vi "AlliGator Save-Load IRFs & Fit Data (Map).vi"(8 "error in (no error)":errorcluster, 9 "Write(T)/Load (F)":bool, 10 "File Path":path, 11 "Data Value Reference in":refnum<data-value>) -> (0 "error out":errorcluster, 3 "Data Value Reference out":refnum<data-value>, 4 "Message":string)   [LabVIEW 2021, in "AlliGator Decay Fit Parameter Map.lvlib"]
doc: "Load/Save Decay Fit Parameter Map & Metadata from/to HDF5 file."
uses:
  AlliGator Decay Fit Parameter Map.lvlib
  Internal Variables/AlliGator Internal Variables v2.ctl
  <vilib>/vision/Image Controls.llb/IMAQ Image.ctl
  Internal Variables/AlliGator Gate Image Set.ctl
  Files/AlliGator FLI Dataset Type.ctl
  Files/AlliGator Data Series Type.ctl
  Dual-Channel Datasets/AlliGator Dataset Channel.ctl
  Settings/AlliGator Gate Arithmetic.ctl
  Source Image/AlliGator Displayed Image.ctl
  Image/Named ROI Description.ctl
  Phasor Graph/AlliGator Decay Metadata v3.ctl
  Decay Analysis/Decay Preprocessing/AlliGator Decay Background Subtraction Info.ctl
  Decay Analysis/Decay Preprocessing/AlliGator Baseline Subtraction Method.ctl
  Graphs/XY Graph/XY Graph Plot Shift Parameters.ctl
  Graphs/XY Graph/XY Graph Plot Shift Method.ctl
  Decay Analysis/Decay Preprocessing/AlliGator Decay Extrapolation Parameters.ctl
  Phasor/Calibration Phasor (m, phi).ctl
  Phasor/Phasor Reference Series.ctl
  Phasor/Phasor Calibration Map v2.ctl
  Phasor/Phasor (g, s).ctl
  Phasor Graph/AlliGator Raw Phasor Plot Data v5.ctl
  Phasor/Phasor Standard Deviation Options.ctl
  Phasor Plot/AlliGator Phasor Multi-Harmonic Data.ctl
  Phasor/Phasor Harmonic Data.ctl
  AlliGator Decay Fit Options & Parameters v4.ctl
  Fits/IRF(X)PSED/Decay Fit Options v4.ctl
  Fits/Decay Convolution/Decay Model.ctl
  Fits/Residual Type.ctl
  Fits/IRF(X)PSED/Fit Weights Type v2.ctl
  Fits/Non-linear Fitting Method v2.ctl
  Fits/Fit Calculation Method.ctl
  Fits/Non-linear Fitting Algorithm.ctl
  Decay Analysis/Decay Fit/AlliGator Decay Fit Parameter Constraints 2.ctl
  Fits/IRF(X)PSED/Decay Fit Parameters In List.ctl
  Fits/IRF(X)PSED/MLE Baseline Offset Type.ctl
  Decay Analysis/Decay Preprocessing/AlliGator Decay Preprocessing Parameters.ctl
  Fits/IRF(X)PSED/Decay Fit Parameters & Derived Quantities List v2.ctl
  Fits/IRF(X)PSED/Decay Fit Result Constraint.ctl
  AlliGator Parameter Maps Data.ctl
  AlliGator IRFs & Fit Data v3.ctl
  Globals, Variables, Constants/AlliGator Globals.vi
  Files/AlliGator Files.lvlib
  Fits/Fits.lvlib
  Globals, Variables, Constants/AlliGator Globals, Variables & Constants.lvlib
  Graphs/XY Graph/XY Graph Add-Ons.lvlib
  Decay Analysis/Decay Preprocessing/AlliGator Decay Preprocessing.lvlib
  Phasor/Phasor.lvlib
  Image/Image.lvlib
  Phasor Graph/AlliGator Phasor Graph.lvlib
  Phasor Plot/AlliGator Phasor Plot.lvlib
  Source Image/AlliGator Source Image.lvlib
  Internal Variables/AlliGator Internal Variables.lvlib
  Decay Analysis/Decay Fit/AlliGator Decay Fit.lvlib
  Settings/AlliGator Settings.lvlib
  Dual-Channel Datasets/AlliGator Dual-Channel Datasets.lvlib
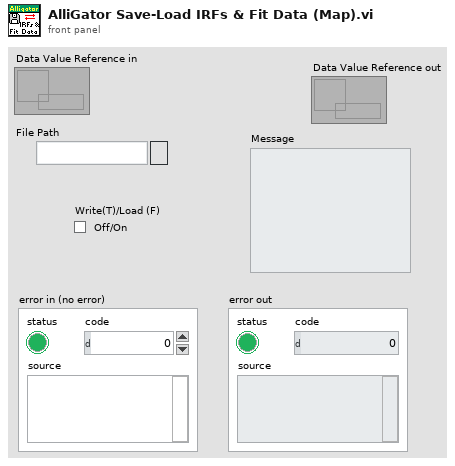
[diagram p1: front panel]
types:
  T1 = typedef "Fits.lvlib/Decay Model.ctl" = enum16{"1-Exponential", "2-Exponentials"}
  T2 = typedef "AlliGator Decay Fit Parameter Map.lvlib/AlliGator IRFs & Fit Data v3.ctl" = cluster{"IRF Array Time Axis":dbl[], "[IRFs]":dbl[][], "[Decay Fit Parameter Names]":T3[], "[Multiple Decays Fit Parameters]":dbl[][], "Fit Options: Decay Preprocessing Parameters":T4, "Fit Options: Reference Decay":cluster{"t Array":dbl[], "I Array":dbl[]}, "[Decay Sum]":dbl[]}
  T3 = typedef "Fits.lvlib/Decay Fit Parameters & Derived Quantities List v2.ctl" = enum16{"Offset", "Baseline", "A_1", "tau_1", "A_2", "tau_2", "<tau>_a", "f1_a", "f2_a", "<tau>_i", "f1_i", "f2_i", "-", "R^2", "Chi^2"}
  T4 = typedef "AlliGator Decay Preprocessing.lvlib/AlliGator Decay Preprocessing Parameters.ctl" = cluster{"Background Subtraction":bool, "Straighten Decay":bool, "Reverse Gates":bool, "1-Normalized Decay":bool, "Smoothen Decay":bool, "Smoothing Parameter":dbl, "Shift Decay":bool, "Decay Shift Parameters":T5, "Extrapolate Decay":bool, "Additional Points":u32, "Head Fraction":dbl, "Pixel-Normalize Decay":bool, "Use Periodicity":bool, "Use Cursors":bool, "Tail Fraction":dbl, "Use Decay Pre-Processing":bool, "Fold Decay":bool, "# Folds":u32, "[0-1]-Normalized Decay":bool}
  T5 = typedef "XY Graph Add-Ons.lvlib/XY Graph Plot Shift Parameters.ctl" = cluster{"Type":T6, "Shift":dbl[unit], "Threshold":dbl, "Rotate":bool}
  T6 = typedef "XY Graph Add-Ons.lvlib/XY Graph Plot Shift Method.ctl" = enum16{"Default", "CFD", "Threshold", "Cross-Correlation"}
  T7 = typedef "AlliGator Internal Variables.lvlib/AlliGator Internal Variables v2.ctl" = cluster{"----------------------------- Images -----------------------------":u8, "Displayed Image":T8, "White Light Image":T8, "Mask Image":T8, "ROI Mask Image":T8, "Current Dataset Images 1":T9, "Background Dataset Images 1":T9, "Current Dataset Images 2":T9, "Background Dataset Images 2":T9, "Current Dataset Arithmetic Images":T9, "Accumulated Dataset Images 1":T9, "Accumulated Dataset Images 2":T9, "Accumulated Dataset Arithmetic Images":T9, "----------------------------- File Paths -----------------------------":u8, "Phasor Plot Image":T8, "Decay Fit Parameter Map Image":T8, "Parameter Map Image":T8, "Single Data Point Path":path, "White Light Image Path":path, "Mask Image Path":path, "Time-Series Folder":path, "[Time-Series Paths]":path[], "----------------------------- FLI Dataset -----------------------------":u8, "Current Dataset":i32, "Single Dataset Type":T10, "Current Folder":string, "AlliGator Data Series Type":T11, "# Datasets":i32, "Dual-Channel Dataset":bool, "Selected Channel Name":string, "Dataset Channel":T12, "Channel Arithmetic":T13, "Dual-Channel Background Dataset":bool, "Background Channel":T12, "Dual-Channel Accumulated Dataset":bool, "Start Time":dbl, "[Time-Series Timestamps]":dbl[], "[Intensity Corrections]":dbl[], "Time Series Script":bool, "Type of Displayed Image":T14, "Gate Image Slide":u16, "# Gates":i32, "ROIs":T15[], "----------------------------- Decays -----------------------------":u8, "ROI Decay":cluster{"t Array":dbl[], "I Array":dbl[]}, "Valid Decay":bool, "Decay  Metadata":T17, "Reference Decay Plot Name":string, "Reference Decay":cluster{"t Array":dbl[], "I Array":dbl[]}, "Decay Shift Plot":cluster{"Time Stamps":dbl[], "Decay Shifts":dbl[]}, "[Decays Max Values]":sgl[], "[Decays Min Values]":sgl[], "----------------------------- Calibration -----------------------------":u8, "Calibration Phasor":T21, "Calibration Phasor Series":T22, "Phasor Calibration Map":T23, "Calibration Map MD5 Digest":string, "----------------------------- Phasor Graph -----------------------------":u8, "Last Raw Phasor":T24, "Last Calibrated Phasor":T24, "Last Calibrated Phasor SDV":T24, "Phasor Graph:Phasor Plot":cluster{"g Array":dbl[], "s Array":dbl[]}, "Phasor Graph:Phasor SDV Plot":cluster{"g Array":dbl[], "s Array":dbl[]}, "[Phasor Graph:Raw Phasor Plots]":T25[], "Phasor Plot locked to Ref 1":i32, "[Phasor Plot(s) locked to Ref 1]":i32[], "[Phasor Plot(s) locked to Ref 2]":i32[], "[Pixel Phasors]":T24[], "----------------------------- Phasor Plot -----------------------------":u8, "[[Sum Image]]":dbl[][], "[[CSG Phasors]]":csg[][], "[[Valid Pixel?]]":bool[][], "[[Phasor Ratios]]":dbl[][], "[[Average Lifetimes]]":dbl[][], "Amplitude Weighted Average Lifetime":bool, "I/m/phi Dataset":cluster{"I/m/phi Dataset?":bool, "Base Frequency":dbl[unit], "Harmonic Orders":u8[]}, "Multi Phasor Plot Data":T27, "----------------------------- Decay Fit Parameter Map -----------------------------":u8, "Decay Fit Options & Parameters":T29, "Fit Options: Decay Preprocessing Parameters":T4, "Fit Options: Reference Decay":cluster{"t Array":dbl[], "I Array":dbl[]}, "Is Full Image Parameters Map":bool, "Is Single-Pixels Parameters Map":bool, "NLSF Parameters Map X Resolution":i32, "NLSF Parameters Map Y Resolution":i32, "[Single Decay Fit Parameters]":dbl[], "Fit Model":T1, "[[Multiple Decays Fit Parameters]]":dbl[][], "[[Multiple Decays Fit Parameter SDVs]]":dbl[][], "[[IRFs]]":dbl[][], "[ROI Descriptors]":T16[], "IRF Array Time Axis":dbl[], "Decay Array Time Axis":dbl[], "[Decay Fit Parameter Names]":T3[], "[Decay Sum]":dbl[], "Array of Decay Fit Result Constraints":T39[], "Selected ROIs Array":bool[], "----------------------------- Parameter Maps -----------------------------":u8, "[Map Set Names]":string[], "[Parameter Maps]":T40[], "[[User-defined Quantities]]":dbl[][], "User-defined Quantity":string}
  T8 = typedef "IMAQ Image.ctl" = refnum<image>
  T9 = typedef "AlliGator Internal Variables.lvlib/AlliGator Gate Image Set.ctl" = cluster{"SGL Image Max":T8, "SGL Image Sum":T8, "SGL Gate Images":T8[], "SGL Image Min":T8}
  T10 = typedef "AlliGator Files.lvlib/AlliGator FLI Dataset Type.ctl" = enum16{"HDF5 FLI Dataset", "Gate Image Folder", ".sdt FLI Dataset (Becker & Hickl)", ".ptu FLI Dataset (PicoQuant)", "SS1 FLI Dataset", "SS2 FLI Dataset", "I/m/phi Dataset", ".bin FLI Dataset (PicoQuant Binned)", ".bin FLI Dataset (Piccolo Binned)", ".mat FLI Dataset"}
  T11 = typedef "AlliGator Files.lvlib/AlliGator Data Series Type.ctl" = enum16{"Not a Supported Series", "Gate Images Folder Series", "SwissSPAD 2 Dataset Series", "B&H FLI Dataset Series", "PicoQuant PTU FLI Dataset Series", "PicoQuant BIN FLI Dataset Series", "Piccolo hist BIN FLI Dataset Series", "HDF5 FLI Dataset Series"}
  T12 = typedef "AlliGator Dual-Channel Datasets.lvlib/AlliGator Dataset Channel.ctl" = enum16{"G2", "INT"}
  T13 = typedef "AlliGator Settings.lvlib/AlliGator Gate Arithmetic.ctl" = enum16{"None", "INT-G2", "G2/INT*<INT>", "(1 - G2/INT)*<INT>"}
  T14 = typedef "AlliGator Source Image.lvlib/AlliGator Displayed Image.ctl" = enum16{"Single Gate", "Sum of All Gates", "Max of All Gates", "Min of All Gates", "-", "White Ligth Image", "Mask Image"}
  T15 = typedef "Image.lvlib/Named ROI Description.ctl" = cluster{"ROI Descriptor":T16, "ROI Name":string, "Overlay Color":u32}
  T16 = typedef "ROI Descriptor" = cluster{"Global Rectangle":i32[], "Contours":cluster{"ID":enum32{"External", "Internal"}, "Type":u32, "Coordinates":i32[]}[]}
  T17 = typedef "AlliGator Phasor Graph.lvlib/AlliGator Decay Metadata v3.ctl" = cluster{"ROI Descriptor":T16, "ROI Center":cluster{"X":i32, "Y":i32}, "Decay Background Subtraction Info":T18, "Decay Reverted":bool, "Decay Smoothened":bool, "Decay Straightened":bool, "Fitted Tau (Decay Straightening)":dbl, "Decay Shift Parameters":T5, "Decay Shifted":bool, "Decay Extrapolated":bool, "Decay Extrapolation Parameters":T20, "Decay Normalized":bool, "Fold Decay":bool, "# Folds":u32}
  T18 = typedef "AlliGator Decay Preprocessing.lvlib/AlliGator Decay Background Subtraction Info.ctl" = cluster{"Laser Period":dbl[unit], "Gate Duration":dbl[unit], "Baseline Subtraction Method":T19, "Background Definition Range":cluster{"Min Gate":dbl[unit], "Max Gate":dbl[unit]}, "Total Intensity w/o Bkgd Subtraction":dbl, "Bkgd-subtracted Intensity (exp)":dbl, "# Data Points":i32, "Background/Gate":dbl, "Fitted Lifetime":dbl[unit], "Bkgd-subtracted Intensity (theo)":dbl}
  T19 = typedef "AlliGator Decay Preprocessing.lvlib/AlliGator Baseline Subtraction Method.ctl" = enum16{"Mean", "Min", "Square Gated Single-Exponential", "File", "Constant"}
  T20 = typedef "AlliGator Decay Preprocessing.lvlib/AlliGator Decay Extrapolation Parameters.ctl" = cluster{"Additional Points":u32, "Head Fraction":dbl, "Fitted Tau":dbl, "Use Periodicity":bool, "Use Cursors":bool, "Tail Fraction":dbl}
  T21 = typedef "Phasor.lvlib/Calibration Phasor (m, phi).ctl" = cluster{"m":dbl, "phi":dbl, "Phasor Frequency":dbl[unit], "Reference Lifetime":dbl[unit]}
  T22 = typedef "Phasor.lvlib/Phasor Reference Series.ctl" = cluster{"m Array":dbl[], "phi Array":dbl[], "Phasor Frequency":dbl[unit], "Calibration Lifetime":dbl[unit]}
  T23 = typedef "Phasor.lvlib/Phasor Calibration Map v2.ctl" = cluster{"Phasor Frequency":dbl[unit], "Calibration Lifetime":dbl[unit], "ROI Centers":cluster{"X":i32, "Y":i32}[], "ROI Descriptors":T16[], "Map Resolution X":i32, "Map Resolution Y":i32, "z Array":cdb[]}
  T24 = typedef "Phasor.lvlib/Phasor (g, s).ctl" = cluster{"g":dbl, "s":dbl}
  T25 = typedef "AlliGator Phasor Graph.lvlib/AlliGator Raw Phasor Plot Data v5.ctl" = cluster{"Phasor Plot Name":string, "Raw Phasor Plot":T24[], "Phasor Frequency":dbl[unit], "[Decay Metadata]":T17[], "Raw Phasor Plot SDV":T24[], "Phasor SDV Options":T26, "[Calibration Phasor]":T21[], "Intensity Array":dbl[]}
  T26 = typedef "Phasor.lvlib/Phasor Standard Deviation Options.ctl" = cluster{"Compute Estimated SDV":bool, "# Replicas":u32, "Use Estimated Average Phasor":bool}
  T27 = typedef "AlliGator Phasor Plot.lvlib/AlliGator Phasor Multi-Harmonic Data.ctl" = cluster{"Base Frequency":dbl[unit], "# Harmonics":u8, "Harmonic Orders":u8[], "Phasor Plot Settings Checksum":u64, "Phasor Harmonic Data Array":T28[]}
  T28 = typedef "Phasor.lvlib/Phasor Harmonic Data.ctl" = cluster{"Phasor Harmonic Name":string, "Phasor Plot Settings Checksum":u64, "Phasor Frequency":dbl[unit], "Base Frequency":dbl[unit], "Harmonic Order":u8, "Phasor Plot Parameters":string, "Phasor Array [[CSG]]":csg[][], "Dataset File Path":path}
  T29 = typedef "AlliGator Decay Fit Parameter Map.lvlib/AlliGator Decay Fit Options & Parameters v4.ctl" = cluster{"SYNC Period":dbl[unit], "Fit Options":T30, "Fit Parameter Constraints":T36[], "MLE Baseline Offset":dbl, "MLE Baseline Offset Type":T38}
  T30 = typedef "Fits.lvlib/Decay Fit Options v4.ctl" = cluster{"Show Fit Residuals":bool, "Fit Model":T1, "Residual Type":T31, "Max Decay Percentile":dbl, "Min Decay Percentile":dbl, "Show Full Decay":bool, "Weights":T32, "Fitting Method":T33, "Compute Parameter Uncertainties":bool, "Periodic Boundaries":bool, "Model Calculation":T34, "Period":dbl[unit], "Termination Criteria":cluster{"Max Iterations":i32, "Max Function Calls":i32, "Max Time":dbl[unit], "Function Tolerance":dbl, "Parameter Tolerance":dbl, "Gradient Tolerance":dbl, "Min Lambda":dbl, "Max Lambda":dbl, "Initial Tick Count":u32}, "Offset Resolution":dbl[unit], "Use Local IRF":bool, "Fitting Algorithm":T35, "Show Confidence Interval ":bool, "Confidence Level":dbl}
  T31 = typedef "Fits.lvlib/Residual Type.ctl" = enum16{"Standard", "Normalized", "Reduced"}
  T32 = typedef "Fits.lvlib/Fit Weights Type v2.ctl" = enum16{"Unweighted", "1/Variance (Neyman)", "1/Variance (Pearson)", "Best of All"}
  T33 = typedef "Fits.lvlib/Non-linear Fitting Method v2.ctl" = enum16{"Least Square", "Least Absolute Residual", "Bisquare", "MLE", "-", "Best of All"}
  T34 = typedef "Fits.lvlib/Fit Calculation Method.ctl" = enum16{"Simulation", "Convolution", "Integration"}
  T35 = typedef "Fits.lvlib/Non-linear Fitting Algorithm.ctl" = enum16{"Levenberg-Marquardt", "Trust-Region Dogleg"}
  T36 = typedef "AlliGator Decay Fit.lvlib/AlliGator Decay Fit Parameter Constraints 2.ctl" = cluster{"Fit Parameter":T37, "Min Value":dbl, "Max Value":dbl, "Global":bool, "Used":bool}
  T37 = typedef "Fits.lvlib/Decay Fit Parameters In List.ctl" = enum16{"Offset", "Baseline", "A_1", "tau_1", "A_2", "tau_2"}
  T38 = typedef "Fits.lvlib/MLE Baseline Offset Type.ctl" = enum32{"Absolute", "Percentage"}
  T39 = typedef "Fits.lvlib/Decay Fit Result Constraint.ctl" = cluster{"Fit Parameter":enum16{"Offset", "Baseline", "A_1", "tau_1", "A_2", "tau_2", "<tau>_a", "f1_a", "f2_a", "<tau>_i", "f1_i", "f2_i", "-", "R^2", "Chi^2", "Max Relative Residual", "<Residual ACF>", "Residual ACF SDV", "tau_2/tau_1"}, "Min Value":dbl, "Max Value":dbl, "Use Constraint":bool}
  T40 = typedef "AlliGator Decay Fit Parameter Map.lvlib/AlliGator Parameter Maps Data.ctl" = cluster{"Map Set Name":string, "[Parameter Names]":string[], "[[Parameters]]":dbl[][], "[[Parameter SDVs]]":dbl[][], "Decay Array Time Axis":dbl[], "[[IRFs]]":dbl[][], "IRF Array Time Axis":dbl[], "X Resolution":i32, "Y Resolution":i32, "Intensity Array":dbl[]}
  T41 = typedef "AlliGator Decay Fit Parameter Map.lvlib/AlliGator IRFs & Fit Data v1.ctl" = cluster{"IRF Array Time Axis":dbl[], "[IRF]":dbl[][], "[Decay Fit Parameter Name]":T3[], "[Multiple Decays Fit Parameters]":dbl[][]}
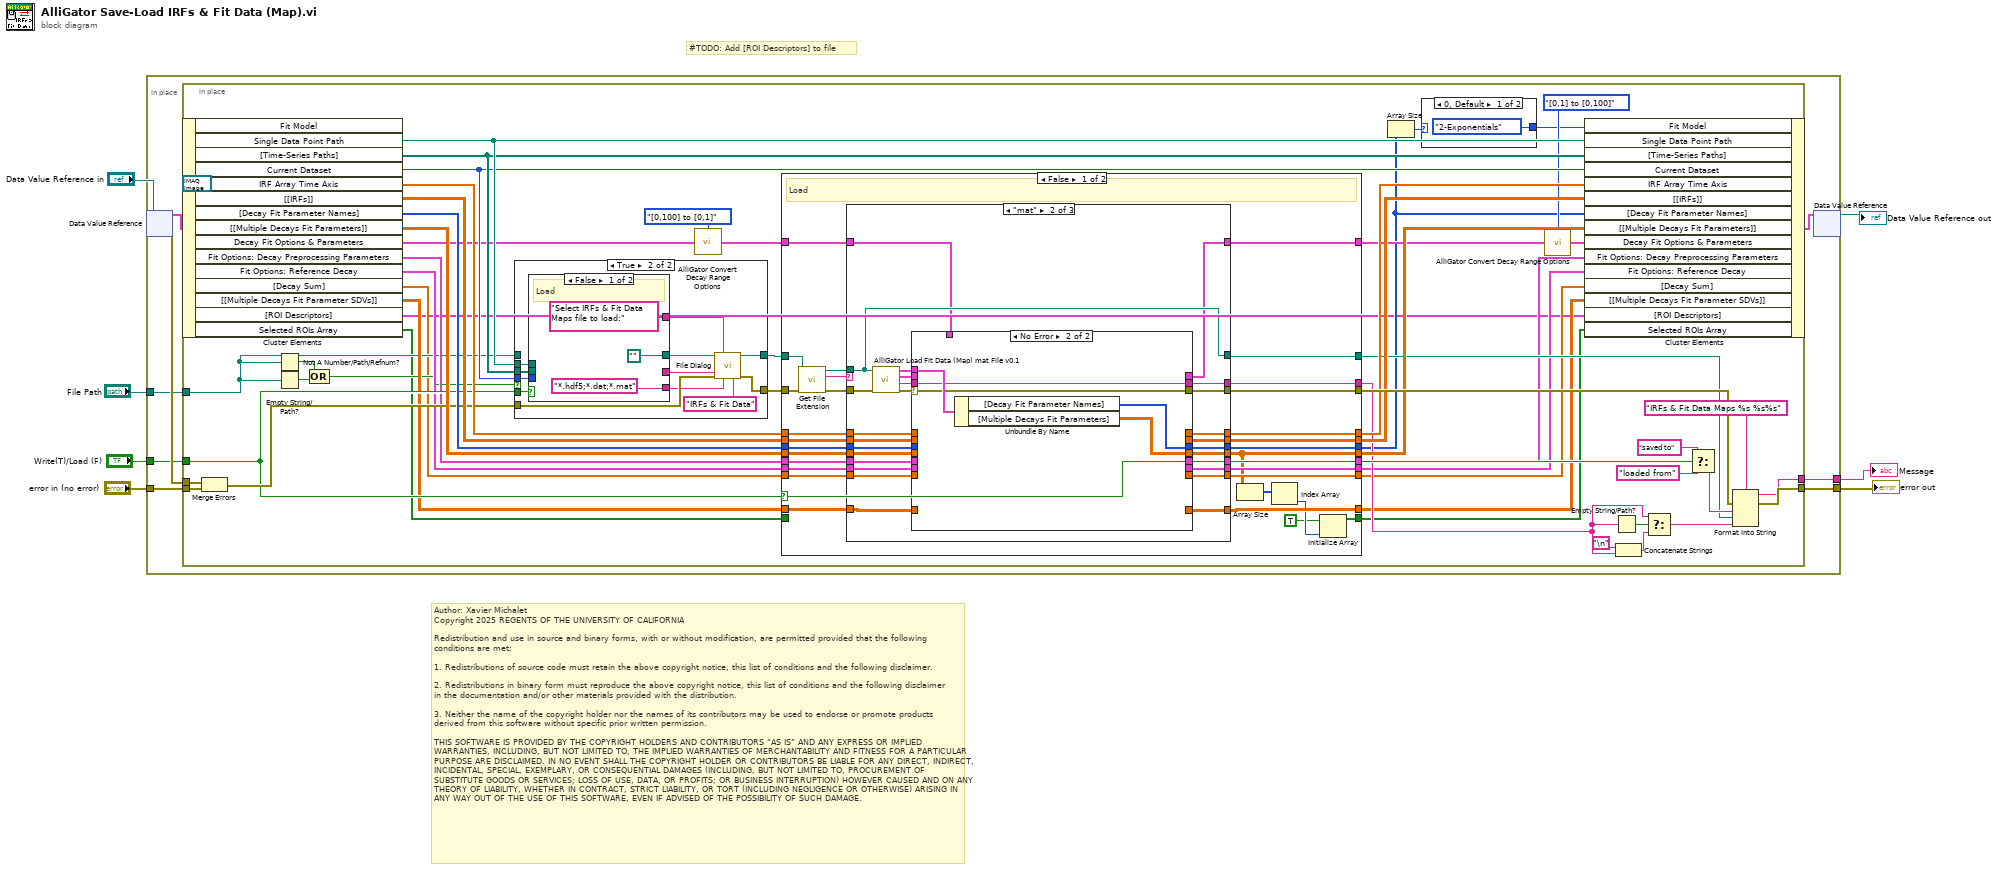
[diagram p0: block diagram]
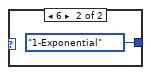
[diagram p2: hidden frame]
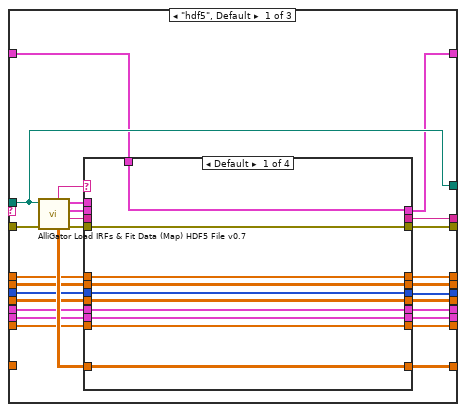
[diagram p3: hidden frame]
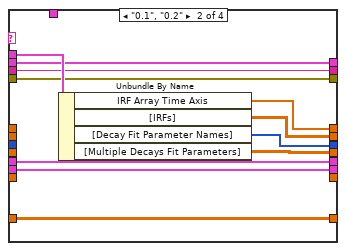
[diagram p4: hidden frame]
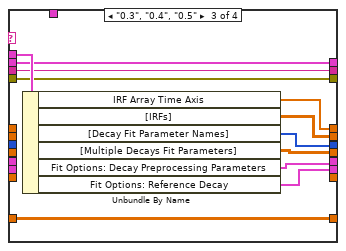
[diagram p5: hidden frame]
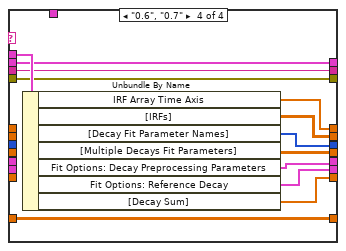
[diagram p6: hidden frame]
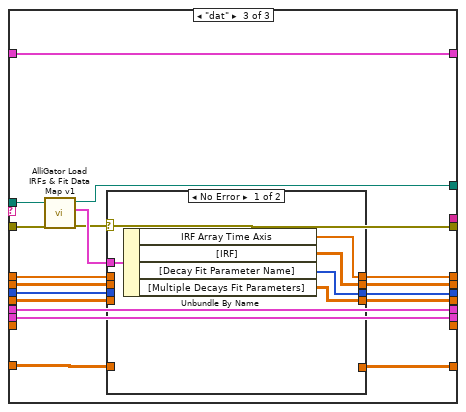
[diagram p8: hidden frame]
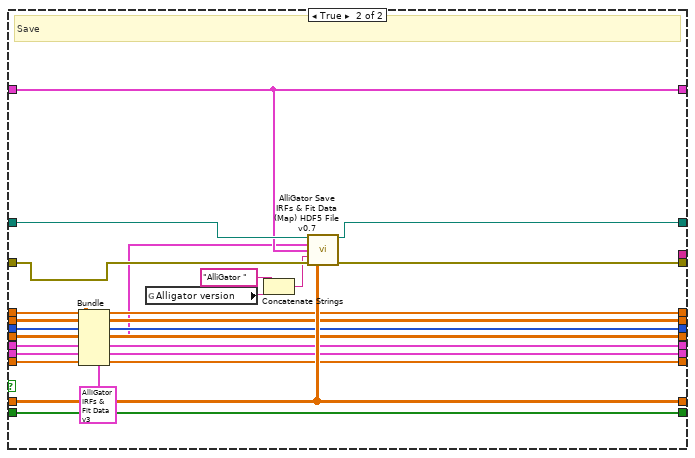
[diagram p10: hidden frame]
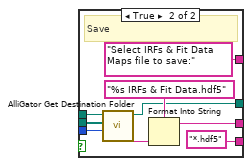
[diagram p12: hidden frame]
diagram:
  # "#TODO: Add [ROI Descriptors] to file"
  # "Author: Xavier Michalet\nCopyright 2025 REGENTS OF THE UNIVERSITY OF CALIFORNIA\n\nRedistribution and use in source and binary forms, with or without modification, are permitted provided that the following conditions are met:\n\n1. Redistributions of source code must retain the above copyright notice, this list of conditions and the following disclaimer.\n\n2. Redistributions in binary form must reproduce the above copyright notice, this list of conditions and the following disclaimer in the documentation and/or other materials provided with the distribution.\n\n3. Neither the name of the copyright holder nor the names of its contributors may be used to endorse or promote products derived from this software without specific prior written permission.\n\nTHIS SOFTWARE IS PROVIDED BY THE COPYRIGHT HOLDERS AND CONTRIBUTORS “AS IS” AND ANY EXPRESS OR IMPLIED WARRANTIES, INCLUDING, BUT NOT LIMITED TO, THE IMPLIED WARRANTIES OF MERCHANTABILITY AND FITNESS FOR A PARTICULAR PURPOSE ARE DISCLAIMED. IN NO EVENT SHALL THE COPYRIGHT HOLDER OR CONTRIBUTORS BE LIABLE FOR ANY DIRECT, INDIRECT, INCIDENTAL, SPECIAL, EXEMPLARY, OR CONSEQUENTIAL DAMAGES (INCLUDING, BUT NOT LIMITED TO, PROCUREMENT OF SUBSTITUTE GOODS OR SERVICES; LOSS OF USE, DATA, OR PROFITS; OR BUSINESS INTERRUPTION) HOWEVER CAUSED AND ON ANY THEORY OF LIABILITY, WHETHER IN CONTRACT, STRICT LIABILITY, OR TORT (INCLUDING NEGLIGENCE OR OTHERWISE) ARISING IN ANY WAY OUT OF THE USE OF THIS SOFTWARE, EVEN IF ADVISED OF THE POSSIBILITY OF SUCH DAMAGE."
  n1 = in-place {
    in-place-border: "error in (no error)" -> [w13]
    in-place-border: [w11] -> w1
    in-place-border: [w10] -> w2
    in-place-border: "Write(T)/Load (F)" -> [w9]
    in-place-border: "File Path" -> [w8]
    n2 = in-place-dvr #1("Data Value Reference in") -> (w15:T7, w12:errorcluster)
    n3 = in-place {
      in-place-border: w13 -> [w68]
      in-place-border: w12 -> [w64]
      in-place-border: [w62] -> w11
      in-place-border: [w61] -> w10
      in-place-border: w9 -> [w43]
      in-place-border: w8 -> [w23]
      (unwired) T8 refnum ("Current Dataset Images.Image Sum")
      n4 = in-place-cluster #2(w15) -> ("Single Data Point Path"=w67:path, "[Time-Series Paths]"=w66:path[], "Current Dataset"=w65:i32, "IRF Array Time Axis"=w56:dbl[], "[[IRFs]]"=w55:dbl[][], "[Decay Fit Parameter Names]"=w54:T3[], "[[Multiple Decays Fit Parameters]]"=w53:dbl[][], "Decay Fit Options & Parameters"=w44:T29, "Fit Options: Decay Preprocessing Parameters"=w35:T4, "Fit Options: Reference Decay"=w34:cluster{"t Array":dbl[], "I Array":dbl[]}, "[Decay Sum]"=w20:dbl[], "[[Multiple Decays Fit Parameter SDVs]]"=w37:dbl[][], "[ROI Descriptors]"=w18:T16[], "Selected ROIs Array"=w17:bool[])  [unwired: 1 out]
      n5 = Merge Errors(w64, w68) -> (w47:errorcluster)
      n6 = Not A Number/Path/Refnum?(number/path/refnum=w23) -> (NaN/Path/Refnum?=w21:bool)
      n7 = Empty String/Path?(string/path=w23) -> (empty?=w48:bool)
      n8 = Compound Arithmetic op=OR(w21, w48) -> (w22:bool)
      n9 = case shown="True" w22 {
        tunnel: w67 -> [_ w273]
        tunnel: w66 -> [_ w272]
        tunnel: w65 -> [_ w271]
        tunnel: w23 -> [w261 _]
        tunnel: w47 -> [w260 w268]
        tunnel: [w261 w267] -> w46
        tunnel: [w260 w266] -> w45
        tunnel: w43 -> [_ w264]
        frame False {
        }
        frame True {
          n10 = case shown="False" w264 {
            tunnel: w273 -> [_ w285]
            tunnel: w272 -> [_ w284]
            tunnel: w271 -> [_ w283]
            tunnel: [path "" w280] -> w270
            tunnel: [_ w279] -> w269
            tunnel: ["Select IRFs & Fit Data Maps file to load:" ("prompt") "Select IRFs & Fit Data Maps file to save:" ("prompt")] -> w263
            tunnel: ["*.hdf5;*.dat;*.mat" ("pattern (all files)") "*.hdf5" ("pattern (all files)")] -> w262
            frame False {
              # "Load"
            }
            frame True {
              # "Save"
              n11 = call "AlliGator Get Destination Folder.vi"("Current Data Set (-1: single)"=w283, "Time-Series Paths"=w284, "Single Data Point Path"=w285) -> ("Data Point Name"=w282:string, "Destination Folder path"=w280:path)  [unwired: 5 in, 2 out]
              n12 = Format Into String(format string="%s IRFs & Fit Data.hdf5", w282) -> (resulting string=w279:string)  [unwired: 2 in, 1 out]
            }
          }
          n13 = call "File Dialog"("start path"=w270, "prompt"=w263, "default name"=w269, "error in"=w268, "pattern (all files)"=w262, "pattern label"="IRFs & Fit Data") -> ("selected path"=w267:path, "error out"=w266:errorcluster)  [unwired: 6 in, 2 out]
        }
      }
      n14 = call "AlliGator Convert Decay Range Options.vi"("Decay Fit Options & Parameters in"=w44, "Percentile Conversion"=enum32{"[0,1] to [0,100]", "[0,100] to [0,1]"}."[0,100] to [0,1]") -> ("Decay Fit Options & Parameters out"=w31:T29)
      n15 = case shown="False" w43 {
        tunnel: [w93 w258] -> w63
        tunnel: [w92 w259] -> w49
        tunnel: w56 -> [w97 w253]
        tunnel: w55 -> [w96 w252]
        tunnel: w54 -> [w95 w251]
        tunnel: w53 -> [w94 w250]
        tunnel: [w100 w253] -> w52
        tunnel: [w99 w252] -> w51
        tunnel: [w98 w251] -> w26
        tunnel: [w75 w250] -> w50
        tunnel: w46 -> [w91 w257]
        tunnel: w45 -> [w89 w256]
        tunnel: w31 -> [w85 w255]
        tunnel: [w86 w255] -> w29
        tunnel: [w84 _] -> w40
        tunnel: w37 -> [w82 w254]
        tunnel: [w83 w254] -> w36
        tunnel: w35 -> [w81 w249]
        tunnel: w34 -> [w79 w248]
        tunnel: [w80 w249] -> w33
        tunnel: [w78 w248] -> w32
        tunnel: w20 -> [w76 w242]
        tunnel: [w77 w242] -> w19
        tunnel: w17 -> [_ w241]
        tunnel: [w71 w241] -> w16
        frame False {
          # "Load"
          n16 = call <vilib>:"Get File Extension.vi"("error in (no error)"=w89, "file"=w91) -> ("error out"=w90:errorcluster, "lowercase file extension"=w88:string, "dup file"=w87:path)  [unwired: 5 in, 2 out]
          n17 = case shown="\"mat\"" w88 {
            tunnel: [w125 w195 w229] -> w100
            tunnel: [w124 w194 w228] -> w99
            tunnel: [w123 w193 w227] -> w98
            tunnel: [w122 w192 w226] -> w75
            tunnel: w97 -> [w107 w179 w225]
            tunnel: w96 -> [w106 w178 w224]
            tunnel: w95 -> [w105 w177 w223]
            tunnel: w94 -> [w104 w176 w222]
            tunnel: [w120 w190 w221] -> w93
            tunnel: [w119 w189 w220] -> w92
            tunnel: w90 -> [w127 w197 w219]
            tunnel: w87 -> [w119 w189 w218]
            tunnel: [w114 w185 w217] -> w86
            tunnel: w85 -> [w103 w175 w217]
            tunnel: [w113 w184 _] -> w84
            tunnel: [w115 w186 w215] -> w83
            tunnel: w82 -> [_ w172 w216]
            tunnel: w81 -> [w111 w183 w214]
            tunnel: [w110 w182 w214] -> w80
            tunnel: w79 -> [w109 w181 w213]
            tunnel: [w108 w180 w213] -> w78
            tunnel: [w102 w174 _] -> w77
            tunnel: w76 -> [w101 w173 _]
            frame "hdf5", Default {
              n18 = call "AlliGator Load IRFs & Fit Data (Map) HDF5 File v0.7.vi"("Error In"=w127, "File Path"=w119) -> ("error out"=w121:errorcluster, "Data Description"=w117:string, "Decay Fit Options & Parameters"=w118:T29, "IRFs & Fit Data Map v3"=w126:T2, "[Multiple Decays Fit Parameters SDV]"=w116:dbl[][], "File Version"=w112:string)  [unwired: 3 in, 1 out]
              n19 = case shown="Default" w112 {
                tunnel: w126 -> [_ w148 w159 w171]
                tunnel: [w137 w147 w158 w170] -> w125
                tunnel: [w136 w146 w157 w169] -> w124
                tunnel: [w135 w145 w156 w168] -> w123
                tunnel: [w134 w144 w155 w167] -> w122
                tunnel: [w130 w143 w154 w166] -> w120
                tunnel: w118 -> [_ w141 w152 w165]
                tunnel: w117 -> [_ w140 w151 w164]
                tunnel: w116 -> [w131 w142 w153 w161]
                tunnel: [w131 w142 w153 w161] -> w115
                tunnel: [w129 w141 w152 w165] -> w114
                tunnel: [_ w140 w151 w164] -> w113
                tunnel: w121 -> [w130 w143 w154 w166]
                tunnel: [w133 w139 w150 w163] -> w110
                tunnel: w111 -> [w133 w139 _ _]
                tunnel: w109 -> [w132 w138 _ _]
                tunnel: [w132 w138 w149 w162] -> w108
                tunnel: w107 -> [w137 _ _ _]
                tunnel: w106 -> [w136 _ _ _]
                tunnel: w105 -> [w135 _ _ _]
                tunnel: w104 -> [w134 _ _ _]
                tunnel: w103 -> [w129 _ _ _]
                tunnel: [w128 _ _ w160] -> w102
                tunnel: w101 -> [w128 _ _ _]
                frame Default {
                }
                frame "0.1", "0.2" {
                  n20 = Unbundle By Name(w148) -> ("IRF Array Time Axis"=w147:dbl[], "[IRFs]"=w146:dbl[][], "[Decay Fit Parameter Names]"=w145:T3[], "[Multiple Decays Fit Parameters]"=w144:dbl[][])
                }
                frame "0.3", "0.4", "0.5" {
                  n21 = Unbundle By Name(w159) -> ("IRF Array Time Axis"=w158:dbl[], "[IRFs]"=w157:dbl[][], "[Decay Fit Parameter Names]"=w156:T3[], "[Multiple Decays Fit Parameters]"=w155:dbl[][], "Fit Options: Decay Preprocessing Parameters"=w150:T4, "Fit Options: Reference Decay"=w149:cluster{"t Array":dbl[], "I Array":dbl[]})
                }
                frame "0.6", "0.7" {
                  n22 = Unbundle By Name(w171) -> ("IRF Array Time Axis"=w170:dbl[], "[IRFs]"=w169:dbl[][], "[Decay Fit Parameter Names]"=w168:T3[], "[Multiple Decays Fit Parameters]"=w167:dbl[][], "Fit Options: Decay Preprocessing Parameters"=w163:T4, "Fit Options: Reference Decay"=w162:cluster{"t Array":dbl[], "I Array":dbl[]}, "[Decay Sum]"=w160:dbl[])
                }
              }
            }
            frame "mat" {
              n23 = call "AlliGator Load Fit Data (Map) mat File v0.1.vi"("Error In"=w197, "File Path"=w189) -> ("error out"=w191:errorcluster, "Data Description"=w187:string, "Decay Fit Options & Parameters"=w188:T29, "IRFs & Fit Data Map v3"=w196:T2)  [unwired: 3 in, 3 out]
              n24 = case shown="No Error" w191 {
                selector: w191 -> [w200 w209]
                tunnel: w196 -> [_ w212]
                tunnel: [w207 _] -> w195
                tunnel: [w206 _] -> w194
                tunnel: [w205 w211] -> w193
                tunnel: [w204 w210] -> w192
                tunnel: [w200 w209] -> w190
                tunnel: w188 -> [_ _]
                tunnel: w187 -> [_ w208]
                tunnel: w172 -> [w201 _]
                tunnel: [w201 _] -> w186
                tunnel: [w199 _] -> w185
                tunnel: [_ w208] -> w184
                tunnel: [w203 _] -> w182
                tunnel: w183 -> [w203 _]
                tunnel: w181 -> [w202 _]
                tunnel: [w202 _] -> w180
                tunnel: w179 -> [w207 _]
                tunnel: w178 -> [w206 _]
                tunnel: w177 -> [w205 _]
                tunnel: w176 -> [w204 _]
                tunnel: w175 -> [w199 _]
                tunnel: [w198 _] -> w174
                tunnel: w173 -> [w198 _]
                frame Error {
                }
                frame No Error {
                  n25 = Unbundle By Name(w212) -> ("[Decay Fit Parameter Names]"=w211:T3[], "[Multiple Decays Fit Parameters]"=w210:dbl[][])
                }
              }
            }
            frame "dat" {
              n26 = call "AlliGator Load IRFs & Fit Data Map v1.vi"("error in (no error)"=w219, "File Path in"=w218) -> ("error out"=w221:errorcluster, "IRFs & Fit  Data Map"=w230:T41, "File Path out"=w220:path)  [unwired: 7 in]
              n27 = case shown="No Error" w221 {
                tunnel: w230 -> [w235 _]
                tunnel: [w234 w240] -> w229
                tunnel: [w233 w239] -> w228
                tunnel: [w232 w238] -> w227
                tunnel: [w231 w237] -> w226
                tunnel: w225 -> [_ w240]
                tunnel: w224 -> [_ w239]
                tunnel: w223 -> [_ w238]
                tunnel: w222 -> [_ w237]
                tunnel: w216 -> [_ w236]
                tunnel: [_ w236] -> w215
                frame No Error {
                  n28 = Unbundle By Name(w235) -> ("IRF Array Time Axis"=w234:dbl[], "[IRF]"=w233:dbl[][], "[Decay Fit Parameter Name]"=w232:T3[], "[Multiple Decays Fit Parameters]"=w231:dbl[][])
                }
                frame Error {
                }
              }
            }
          }
          n29 = Array Size(array=w75) -> (size(s)=w74:i32[])
          n30 = Index Array(array=w74) -> (element=w73:i32)  [unwired: 1 in]
          n31 = Initialize Array(TRUE, w73) -> (w71:bool[])
        }
        frame True {
          # "Save"
          n32 = Bundle(cluster=T2 {"IRF Array Time Axis"=[], "[IRFs]"=[], "[Decay Fit Parameter Names]"=[], "[Multiple Decays Fit Parameters]"=[], "Fit Options: Decay Preprocessing Parameters"={"Background Subtraction"=FALSE, "Straighten Decay"=FALSE, "Reverse Gates"=FALSE, "1-Normalized Decay"=FALSE, "Smoothen Decay"=FALSE, "Smoothing Parameter"=0.0, "Shift Decay"=FALSE, "Decay Shift Parameters"={"Type"=enum."Default", "Shift"=0.0, "Threshold"=0.0, "Rotate"=FALSE}, "Extrapolate Decay"=FALSE, "Additional Points"=0, "Head Fraction"=0.0, "Pixel-Normalize Decay"=FALSE, "Use Periodicity"=FALSE, "Use Cursors"=FALSE, "Tail Fraction"=0.0, "Use Decay Pre-Processing"=FALSE, "Fold Decay"=FALSE, "# Folds"=0, "[0-1]-Normalized Decay"=FALSE}, "Fit Options: Reference Decay"={"t Array"=[], "I Array"=[]}, "[Decay Sum]"=[]} ("output cluster"), "IRF Array Time Axis"=w253, "[IRFs]"=w252, "[Decay Fit Parameter Names]"=w251, "[Multiple Decays Fit Parameters]"=w250, "Fit Options: Decay Preprocessing Parameters"=w249, "Fit Options: Reference Decay"=w248, "[Decay Sum]"=w242) -> (w243:T2)
          n33 = global read "AlliGator Globals.vi" "Alligator version"() -> (w247:string)
          n34 = Concatenate Strings("AlliGator " ("string"), w247) -> (w245:string)
          n35 = call "AlliGator Save IRFs & Fit Data (Map) HDF5 File v0.7.vi"("File Path"=w257, "IRFs & Fit Data Map v3"=w243, "Decay Fit Options & Parameters v3"=w255, "Software + Version"=w245, "Error In"=w256, "[Multiple Decays Fit Parameters SDV]"=w254) -> ("File Path out"=w259:path, "Error Out"=w258:errorcluster)  [unwired: 7 in, 1 out]
        }
      }
      n36 = Array Size(array=w26) -> (size(s)=w25:i32)
      n37 = case shown="0, Default" w25 {
        tunnel: [Decay_Model."2-Exponentials" ("Fit Model") Decay_Model."1-Exponential" ("Fit Model")] -> w24
        frame 0, Default {
        }
        frame 6 {
        }
      }
      n38 = call "AlliGator Convert Decay Range Options.vi"("Decay Fit Options & Parameters in"=w29, "Percentile Conversion"=enum32{"[0,1] to [0,100]", "[0,100] to [0,1]"}."[0,1] to [0,100]") -> ("Decay Fit Options & Parameters out"=w28:T29)
      n39 = in-place-cluster #2("Fit Model"=w24, "Single Data Point Path"=w67, "[Time-Series Paths]"=w66, "Current Dataset"=w65, "IRF Array Time Axis"=w52, "[[IRFs]]"=w51, "[Decay Fit Parameter Names]"=w26, "[[Multiple Decays Fit Parameters]]"=w50, "Decay Fit Options & Parameters"=w28, "Fit Options: Decay Preprocessing Parameters"=w33, "Fit Options: Reference Decay"=w32, "[Decay Sum]"=w19, "[[Multiple Decays Fit Parameter SDVs]]"=w36, "[ROI Descriptors]"=w18, "Selected ROIs Array"=w16) -> (w14:T7)
      n40 = Empty String/Path?(string/path=w40) -> (empty?=w42:bool)
      n41 = Concatenate Strings("\n", w40) -> (w38:string)
      n42 = Select(t=w40, s=w42, f=w38) -> (s? t:f=w41:string)
      n43 = Select(t="saved to" ("format string"), s=w43, f="loaded from" ("format string")) -> (s? t:f=w57:string)
      n44 = Format Into String(format string="IRFs & Fit Data Maps %s %s%s", error in=w63, w57, w49, w41) -> (resulting string=w61:string, error out=w62:errorcluster)  [unwired: 1 in]
    }
    n45 = in-place-dvr #1(w14) -> (→"Data Value Reference out":refnum<data-value>)  [unwired: 1 out]
  }
  "error out" <- w1
  "Message" <- w2
